vi "Encoder.vi"() -> ()   [LabVIEW 2014]
uses:
  <vilib>/Instr/_visa.llb/VISA Set IO Buffer Mask.ctl
  <vilib>/Instr/_visa.llb/VISA Configure Serial Port (Instr).vi
panel:
  out "return count":u32
  in  "write buffer":string
  in  "Boolean":bool
  out "Angle":i8[](graph)
  in  "VISA resource name":refnum<visa-resource-name>
  in  "stop":bool
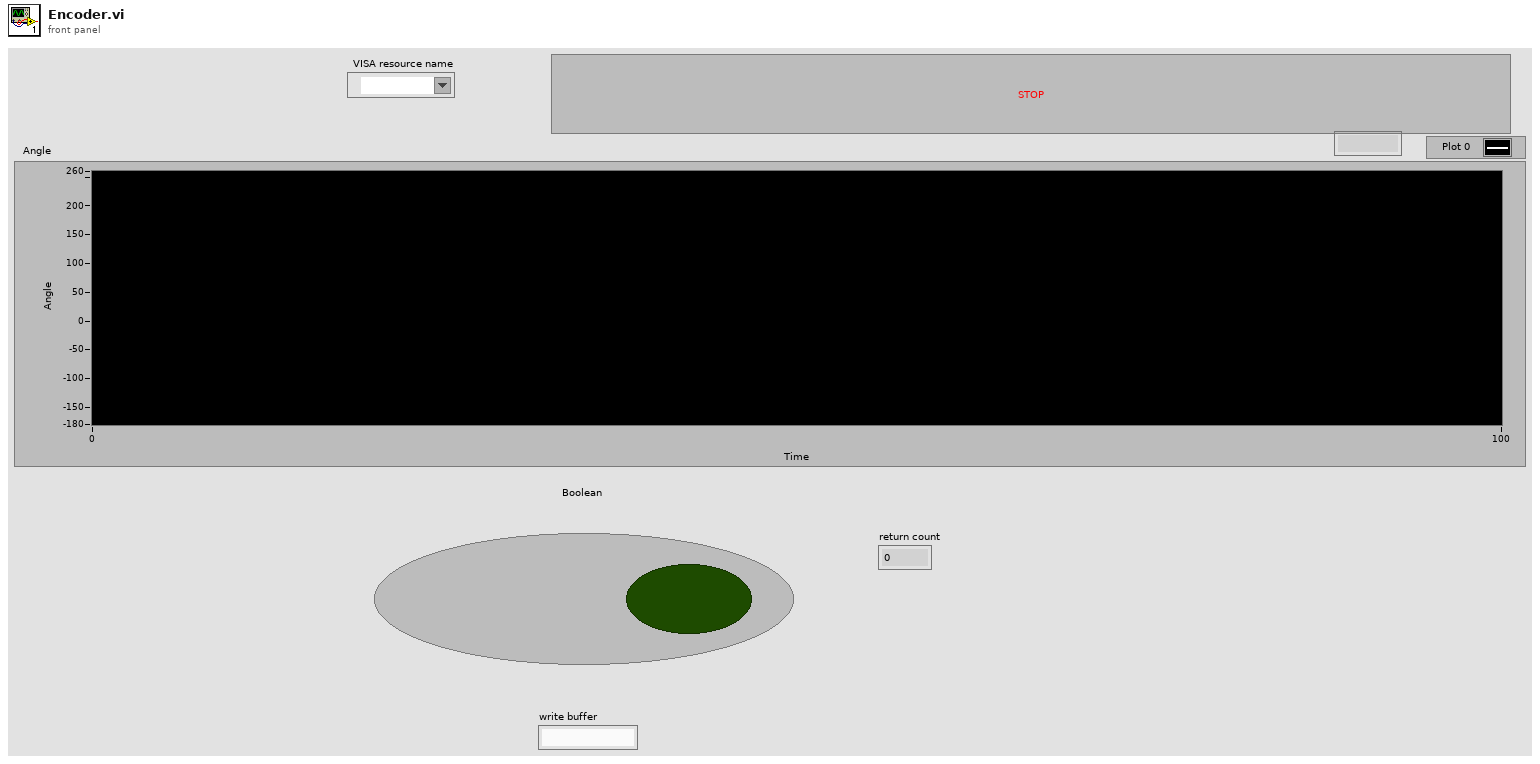
[diagram p1: front panel]
types:
  T1 = typedef "VISA Set IO Buffer Mask.ctl" = u16
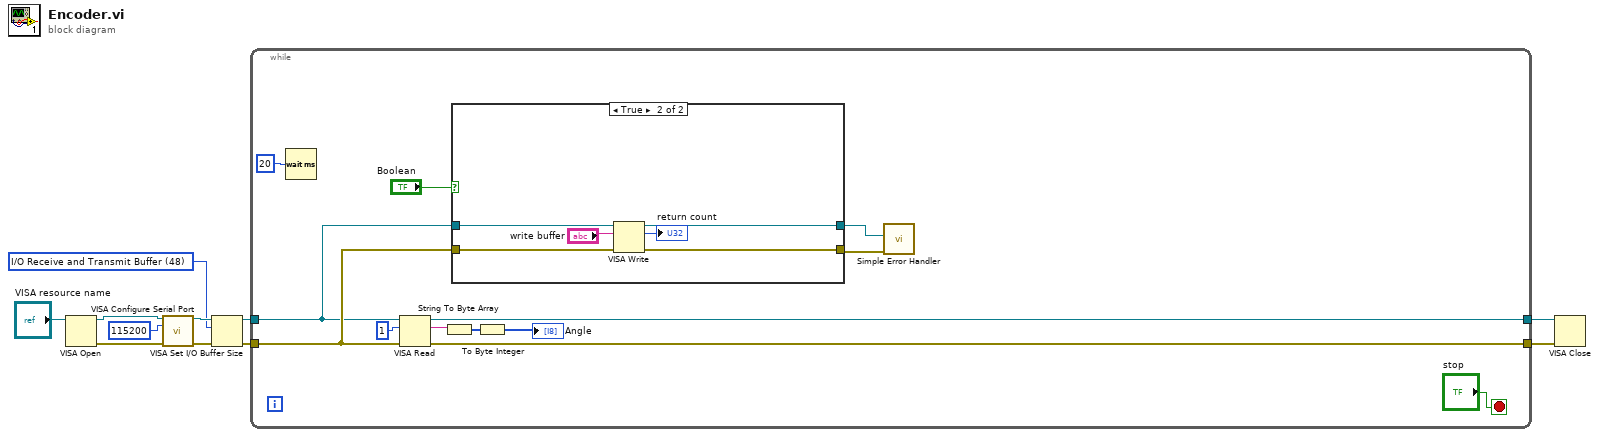
[diagram p0: block diagram]
diagram:
  w7 = T1 48 items=["I/O Receive Buffer"=16, "I/O Transmit Buffer"=32, "I/O Receive and Transmit Buffer"=48] ("Mask")
  n1 = VISA Open(VISA resource name="VISA resource name") -> (VISA resource name=w11:refnum<visa-resource-name>, error out=w8:errorcluster)  [unwired: 4 in]
  n2 = call-poly "VISA Configure Serial Port"("VISA resource name"=w11, "baud rate (9600)"=u32 115200, "error in (no error)"=w8) -> ("VISA resource name out"=w10:refnum<visa-resource-name>, "error out"=w9:errorcluster)  [unwired: 11 in]
  n3 = VISA Set I/O Buffer Size(VISA resource name=w10, mask (16)=w7, error in (no error)=w9) -> (VISA resource name out=w5:refnum<visa-resource-name>, error out=w4:errorcluster)  [unwired: 1 in]
  n4 = while {
    tunnel: w5 -> [w14]
    tunnel: w4 -> [w15]
    tunnel: [w20] -> w2
    tunnel: [w21] -> w1
    stop <- "stop" stop-if-true
    n5 = Wait (ms)(milliseconds to wait=u32 20) -> ()  [unwired: 1 out]
    n6 = VISA Read(VISA resource name=w14, byte count=u32 1, error in (no error)=w15) -> (VISA resource name out=w20:refnum<visa-resource-name>, read buffer=w19:string, error out=w21:errorcluster)  [unwired: 1 out]
    n7 = String To Byte Array(string=w19) -> (unsigned byte array=w18:u8[])
    n8 = case shown="True" "Boolean" {
      tunnel: w15 -> [w25 w32]
      tunnel: w14 -> [w26 w31]
      tunnel: [w25 w30] -> w13
      tunnel: [w26 w29] -> w12
      frame False {
      }
      frame True {
        n9 = VISA Write(VISA resource name=w31, write buffer="write buffer", error in (no error)=w32) -> (VISA resource name out=w29:refnum<visa-resource-name>, return count=→"return count":u32, error out=w30:errorcluster)
      }
    }
    n10 = To Byte Integer(number=w18) -> (8bit integer=→"Angle":i8[])
    n11 = call <vilib>:"Simple Error Handler.vi"("error source (\" \")"=w12, "error in (no error)"=w13) -> ()  [unwired: 3 in, 5 out]
  }
  n12 = VISA Close(VISA resource name=w2, error in (no error)=w1) -> ()  [unwired: 1 out]
